vi "do_stuff.vi"(10 "live data in":dbl[](array[numeric]), 11 "data bus in":dbl[](array[numeric])) -> (2 "live data out":dbl[](array[numeric]), 3 "data bus out":dbl[](array[numeric]))   [LabVIEW 2024, in "IPE Optimization Tester.lvlib"]
uses:
  IPE Optimization Tester.lvlib
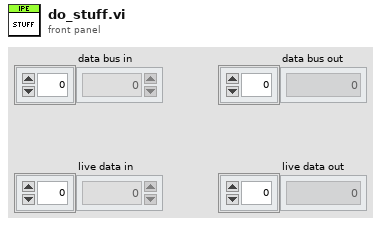
[diagram p1: front panel]
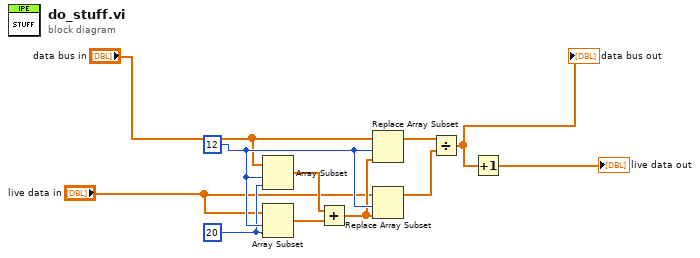
[diagram p0: block diagram]
diagram:
  w3 = 20 ("length")
  w7 = 12 ("index")
  n1 = Array Subset(array="data bus in", index=w7, length=w3) -> (w5:dbl[])
  n2 = Array Subset(array="live data in", index=w7, length=w3) -> (w4:dbl[])
  n3 = Add(x=w5, y=w4) -> (x+y=w6:dbl[])
  n4 = Replace Array Subset(array="data bus in", new element=w6, index=w7) -> (w8:dbl[])
  n5 = Replace Array Subset(array="live data in", new element=w6, index=w7) -> (w9:dbl[])
  n6 = Divide(x=w8, y=w9) -> (x/y=w10:dbl[])
  "data bus out" <- w10
  n7 = Increment(x=w10) -> (x+1=→"live data out":dbl[])
